vi "Write Double.vi"(7 "Channel Index":i32, 8 "error in (no error)":errorcluster, 10 "Data":dbl, 11 "CIFCorePlugin in":refnum<class "CIFCorePlugin.lvclass">) -> (0 "error out":errorcluster, 3 "CIFCorePlugin out":refnum<class "CIFCorePlugin.lvclass">)   [LabVIEW 2021, in "CIFCorePlugin.lvclass"]
uses:
  CIFCorePlugin.lvclass
  CIFCorePlugin.lvclass/CIFCorePlugin.ctl
  Channels/CIFChannelMng/CIFChannelMng.lvclass/CIFChannelMng.ctl
  Channels/CIFChannelMng/Accessors/Read Channel Array.vi
  Channels/CIFChannelMng/Accessors/Write Channel Array.vi
  Channels/CIFChannels/CIFChannels.lvclass
  Channels/CIFChannelMng/CIFChannelMng.lvclass
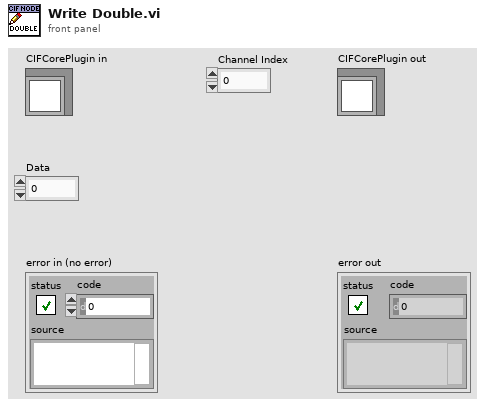
[diagram p1: front panel]
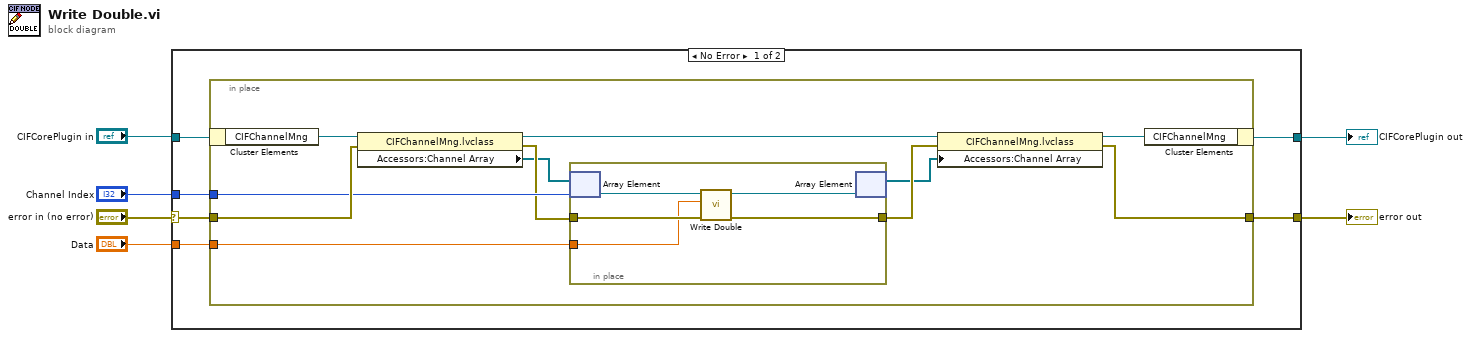
[diagram p0: block diagram]
diagram:
  n1 = case shown="No Error" "error in (no error)" {
    selector: "error in (no error)" -> [w12 w30]
    tunnel: [w11 w30] -> w3
    tunnel: [w8 w29] -> w4
    tunnel: "CIFCorePlugin in" -> [w9 w29]
    tunnel: "Data" -> [w10 _]
    tunnel: "Channel Index" -> [w7 _]
    frame No Error {
      n2 = in-place {
        in-place-border: w12 -> [w20]
        in-place-border: [w13] -> w11
        in-place-border: w10 -> [w23]
        in-place-border: w7 -> [w19]
        n3 = in-place-cluster #1(w9) -> ("CIFChannelMng"=w22:refnum<class "CIFChannelMng.lvclass">)
        n4 = property class="CIFChannelMng.lvclass"(reference=w22, error in=w20) -> (reference out=w18:refnum<class "CIFChannelMng.lvclass">, error out=w17:errorcluster, "Accessors:Channel Array"=w15:refnum<class "CIFChannels.lvclass">[])
        n5 = in-place {
          in-place-border: w17 -> [w27]
          in-place-border: [w26] -> w16
          in-place-border: w23 -> [w24]
          n6 = in-place-array #2(w15, w19) -> (w28:refnum<class "CIFChannels.lvclass">)
          n7 = call-dynamic "Write Double.vi"("error in (no error)"=w27, "Data"=w24, "CIFChannels in"=w28) -> ("error out"=w26:errorcluster, "CIFChannels out"=w25:refnum<class "CIFChannels.lvclass">)  [unwired: 6 in, 1 out]
          n8 = in-place-array #2(w25) -> (w14:refnum<class "CIFChannels.lvclass">[])  [unwired: 1 out]
        }
        n9 = property class="CIFChannelMng.lvclass"(reference=w18, error in=w16, "Accessors:Channel Array"=w14) -> (reference out=w21:refnum<class "CIFChannelMng.lvclass">, error out=w13:errorcluster)
        n10 = in-place-cluster #1("CIFChannelMng"=w21) -> (w8:refnum<class "CIFCorePlugin.lvclass">)
      }
    }
    frame Error {
    }
  }
  "error out" <- w3
  "CIFCorePlugin out" <- w4
